vi "Voltage Read Single.vi"(8 "error in":errorcluster, 9 "Channel Index":i32=1, 11 "Power Supply In":refnum<class "Power Supply.lvclass">) -> (0 "error out":errorcluster, 1 "Changed or First Call?":bool, 2 "Voltage.chX.SP":dbl, 3 "Power Supply Out":refnum<class "Power Supply.lvclass">)   [LabVIEW 2023, in "Power Supply.lvclass"]
uses:
  Power Supply.lvclass
  Power Supply.lvclass/Power Supply.ctl
  Low Level Capabilities/Voltage/Voltage Setpoint/Voltage Setpoint.lvclass
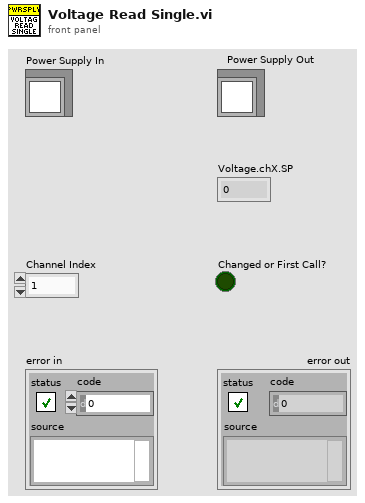
[diagram p1: front panel]
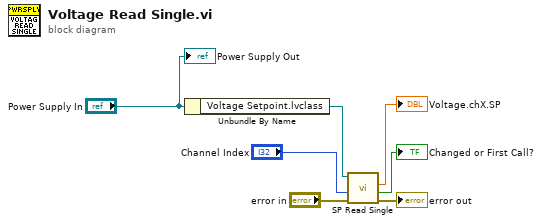
[diagram p0: block diagram]
diagram:
  n1 = Unbundle By Name("Power Supply In") -> ("Voltage Setpoint.lvclass"=w1:refnum<class "Voltage Setpoint.lvclass">)
  n2 = call-dynamic "SP Read Single.vi"("error in"="error in", "Channel Index"="Channel Index", "Voltage Setpoint in"=w1) -> ("error out"=→"error out":errorcluster, "Changed or First Call?"=→"Changed or First Call?":bool, "Current Setpoint"=→"Voltage.chX.SP":dbl)  [unwired: 5 in, 1 out]
  "Power Supply Out" <- "Power Supply In"
